vi "ImpedanceControl.vi"() -> ()   [LabVIEW 2018]
uses:
  <vilib>/Analysis/3filter.llb/Filter Passband Type.ctl
  <vilib>/DAQmx/write.llb/DAQmx Write (Analog DBL 1Chan 1Samp).vi
  <vilib>/DAQmx/read.llb/DAQmx Read (Analog 1D DBL NChan 1Samp).vi
  <vilib>/DAQmx/create/channels.llb/DAQmx Create Channel (AI-Voltage-Basic).vi
  <vilib>/DAQmx/create/channels.llb/DAQmx Create Channel (AO-Voltage-Basic).vi
  <vilib>/DAQmx/miscellaneous.llb/DAQmx Fill In Error Info.vi
  <vilib>/ptbypt/NI_PtbyPt.lvlib
  <vilib>/Analysis/NI_AALBase.lvlib
panel:
  out "Vel Measured":dbl(graph)
  out "Force Measurement":dbl(graph)
  in  "B":dbl min=0.0 step=0.01
  in  "K":dbl min=0.0 step=0.1
  in  "Wall Y/N":bool
  in  "Filter V y/n":bool
  in  "Filter P y/n":bool
  out "Output Voltage":dbl(graph)
  out "Position measurement":dbl(graph)
  in  "Gravity":bool
  in  "Friction":bool
  out "Measurements":dynamicdata(graph)
  in  "stop":bool
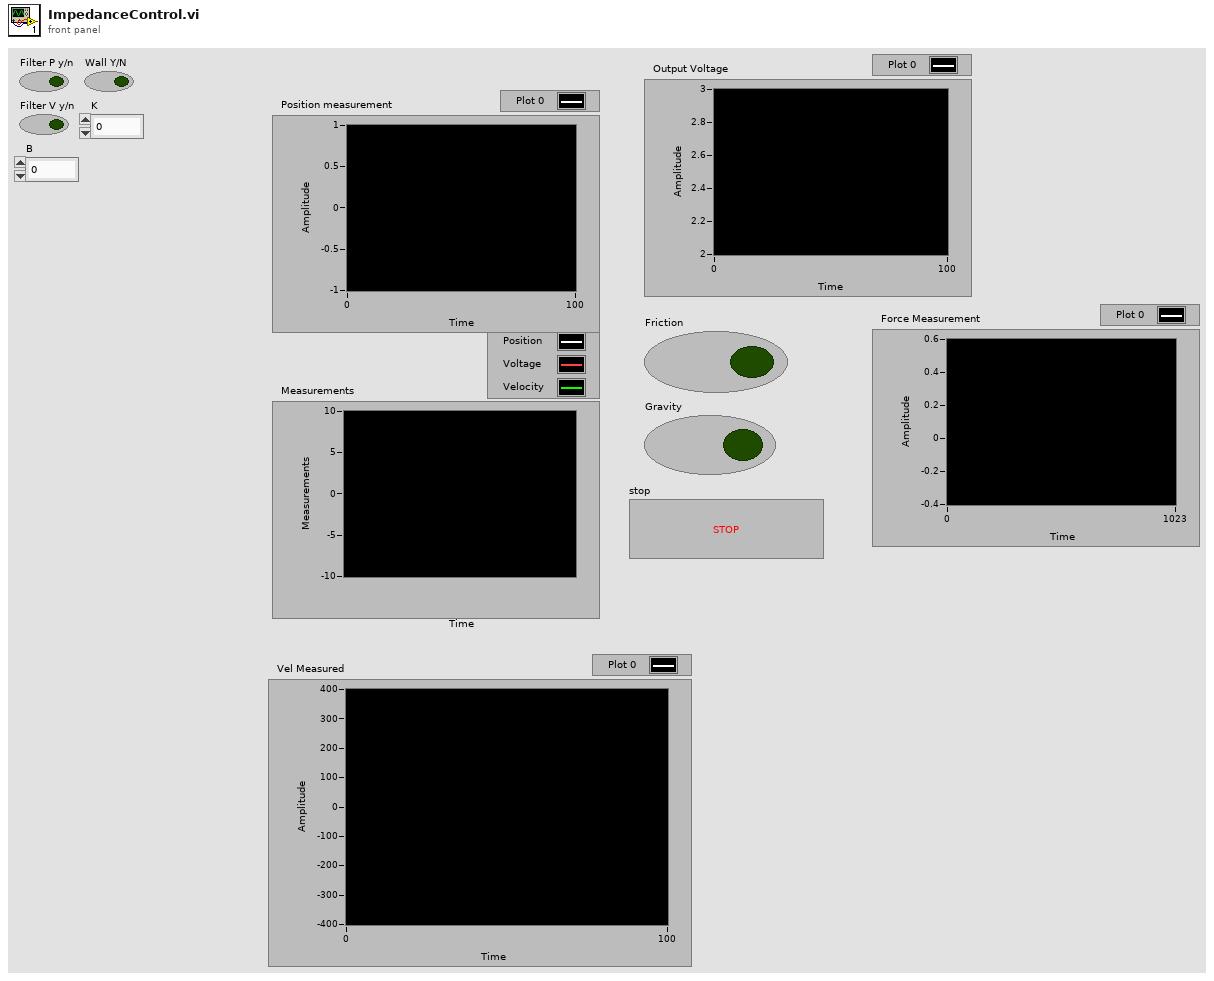
[diagram p1: front panel]
types:
  T1 = typedef "NI_AALBase.lvlib/Filter Passband Type.ctl" = enum32{"Lowpass", "Highpass", "Bandpass", "Bandstop"}
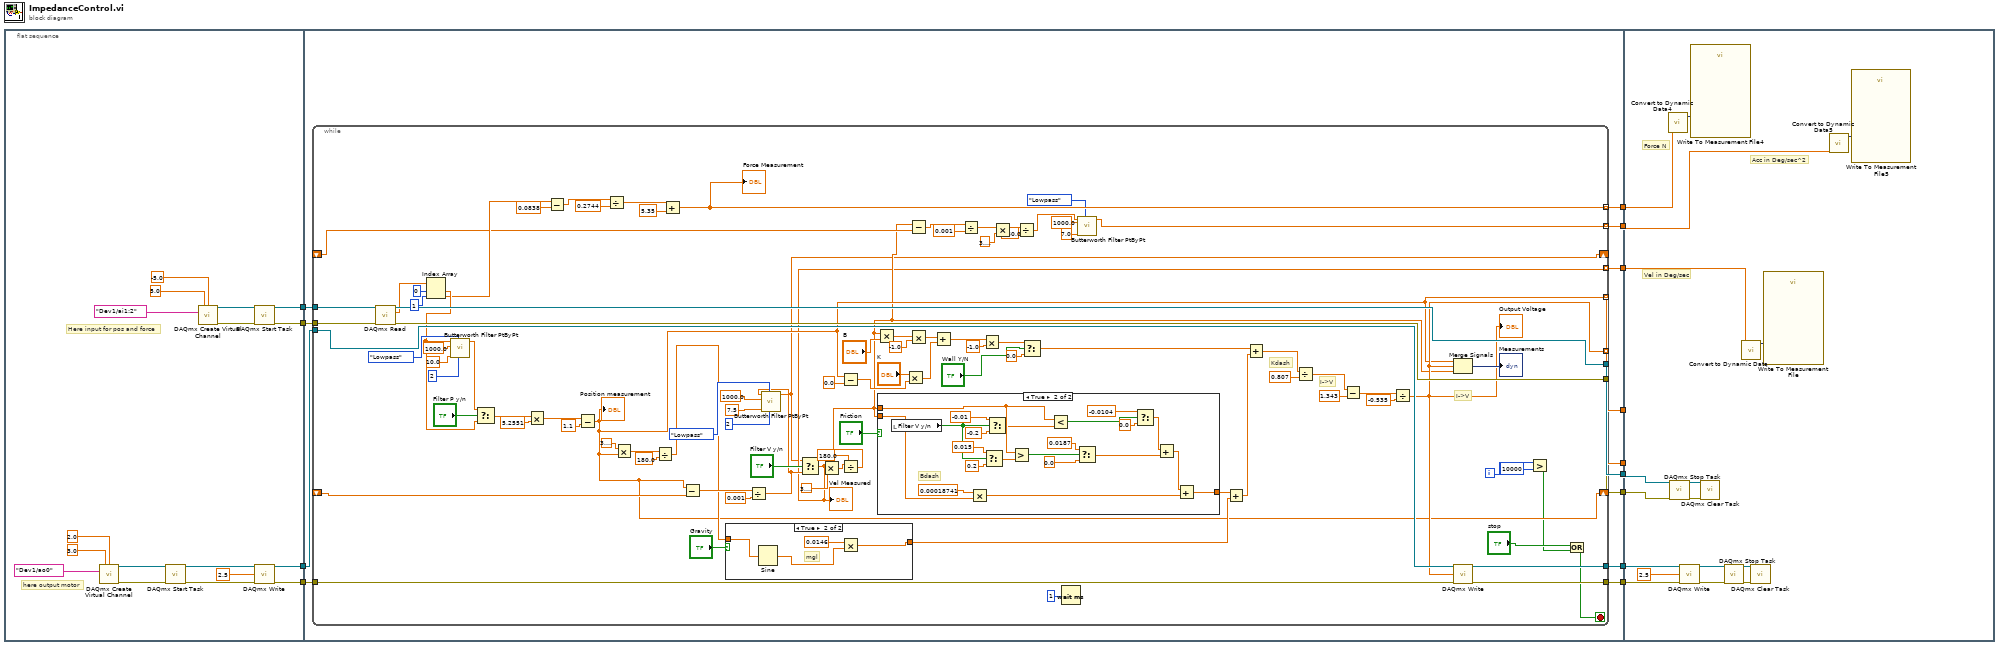
[diagram p0: block diagram]
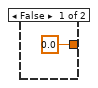
[diagram p2: hidden frame]
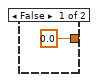
[diagram p3: hidden frame]
diagram:
  n1 = flat-sequence {
    tunnel: [w26] -> w12
    tunnel: [w25] -> w10
    tunnel: [w20] -> w9
    tunnel: [w18] -> w7
    tunnel: [w42] -> w13
    tunnel: w12 -> [w43]
    tunnel: [w40] -> w11
    tunnel: w10 -> [w41]
    tunnel: w9 -> [w39]
    tunnel: [w38] -> w8
    tunnel: w7 -> [w37]
    tunnel: [w36] -> w6
    tunnel: [w35] -> w5
    tunnel: [w34] -> w4
    tunnel: [w33] -> w3
    tunnel: [w32] -> w2
    tunnel: [w31] -> w1
    tunnel: w13 -> [w181]
    tunnel: w11 -> [w178]
    tunnel: w8 -> [w174]
    tunnel: w6 -> [w172]
    tunnel: w5 -> [_]
    tunnel: w4 -> [_]
    tunnel: w3 -> [w170]
    tunnel: w2 -> [w168]
    tunnel: w1 -> [w166]
    frame #0 {
      # "here output motor"
      # "Here input for pos and force"
      n2 = call-poly <vilib>:"DAQmx Create Virtual Channel.vi"("maximum value"=3.0, "minimum value"=2.0, "physical channels"=tag "Dev1/ao0") -> ("task out"=w30:refnum<k21>, "error out"=w29:errorcluster)  [unwired: 11 in]
      n3 = call <vilib>:"DAQmx Start Task.vi"("task/channels in"=w30, "error in"=w29) -> ("task out"=w28:refnum<k21>, "error out"=w27:errorcluster)  [unwired: 12 in]
      n4 = call-poly <vilib>:"DAQmx Create Virtual Channel.vi"("maximum value"=5.0, "minimum value"=-5.0, "physical channels"=tag "Dev1/ai1:2") -> ("task out"=w21:refnum<k21>, "error out"=w19:errorcluster)  [unwired: 11 in]
      n5 = call <vilib>:"DAQmx Start Task.vi"("task/channels in"=w21, "error in"=w19) -> ("task out"=w20:refnum<k21>, "error out"=w18:errorcluster)  [unwired: 12 in]
      n6 = call-poly <vilib>:"DAQmx Write.vi"("task/channels in"=w28, "data"=2.5, "error in"=w27) -> ("task out"=w26:refnum<k21>, "error out"=w25:errorcluster)  [unwired: 10 in, 1 out]
    }
    frame #1 {
      n7 = while {
        tunnel: w43 -> [w137]
        tunnel: [w136] -> w42
        tunnel: w41 -> [w135]
        tunnel: [w134] -> w40
        tunnel: w39 -> [w133]
        tunnel: [w132] -> w38
        tunnel: w37 -> [w131]
        tunnel: [w130] -> w36
        tunnel: [w65] -> w35 mode=indexing
        tunnel: [w101] -> w34 mode=indexing
        shift-right: [w65] -> _
        shift-left: _ -> [w122]
        tunnel: [w64] -> w33 mode=indexing
        shift-right: [w49] -> _
        shift-left: _ -> [w74]
        tunnel: [w53] -> w32 mode=indexing
        tunnel: [w59] -> w31 mode=indexing
        i -> [w57]
        stop <- w54 stop-if-true
        # "I->V"
        # "I->V"
        # "Kdash"
        n8 = call-poly <vilib>:"DAQmx Read.vi"("task/channels in"=w133, "error in"=w131) -> ("task out"=w132:refnum<k21>, "data"=w84:dbl[], "error out"=w130:errorcluster)  [unwired: 11 in]
        n9 = Index Array(array=w84, index #1=0 ("index"), index #2=1 ("index")) -> (element #1=w81:dbl, element #2=w80:dbl)
        n10 = call <vilib>:"Butterworth Filter PtByPt.vi"("order"=2, "filter type"=Filter_Passband_Type."Lowpass", "low cutoff freq: fl"=10.0, "sampling freq: fs"=1000.0, "x"=w81) -> ("Filtered x"=w99:dbl)  [unwired: 4 in, 1 out]
        n11 = Select(t=w99, s="Filter P y/n", f=w81) -> (s? t:f=w93:dbl)
        n12 = Multiply(x=w93, y=5.2551) -> (x*y=w123:dbl)
        n13 = Subtract(x=w80, y=0.0838) -> (x-y=w78:dbl)
        n14 = Subtract(x=w123, y=1.1) -> (x-y=w65:dbl)
        "Position measurement" <- w65
        n15 = Divide(x=w78, y=0.2744) -> (x/y=w76:dbl)
        n16 = Multiply(x=3.141592653589793, y=w65) -> (x*y=w105:dbl)
        n17 = Divide(x=w105, y=180.0) -> (x/y=w70:dbl)
        n18 = Add(x=w76, y=5.35) -> (x+y=w64:dbl)
        "Force Measurement" <- w64
        n19 = Subtract(x=w65, y=w122) -> (x-y=w116:dbl)
        n20 = case shown="True" "Gravity" {
          tunnel: [0.0 w164] -> w117
          tunnel: w70 -> [_ w161]
          frame False {
          }
          frame True {
            # "mgl"
            n21 = Sine(x=w161) -> (sin(x)=w163:dbl)
            n22 = Multiply(x=0.0146, y=w163) -> (x*y=w164:dbl)
          }
        }
        n23 = Divide(x=w116, y=0.001) -> (x/y=w85:dbl)
        n24 = call <vilib>:"Butterworth Filter PtByPt.vi"("order"=2, "filter type"=Filter_Passband_Type."Lowpass", "low cutoff freq: fl"=7.5, "sampling freq: fs"=1000.0, "x"=w85) -> ("Filtered x"=w49:dbl)  [unwired: 4 in, 1 out]
        n25 = Select(t=w49, s="Filter V y/n", f=w85) -> (s? t:f=w59:dbl)
        "Vel Measured" <- w59
        n26 = Multiply(x=w59, y=3.141592653589793) -> (x*y=w62:dbl)
        n27 = Subtract(x=w65, y=0.0) -> (x-y=w89:dbl)
        n28 = Divide(x=w62, y=180.0) -> (x/y=w60:dbl)
        n29 = Multiply(x=w60, y="B") -> (x*y=w68:dbl)
        n30 = case shown="True" "Friction" {
          tunnel: w60 -> [_ w159]
          tunnel: [0.0 w150] -> w118
          tunnel: w60 -> [_ w149]
          frame False {
          }
          frame True {
            # "Bdash"
            n31 = local read "Filter V y/n"() -> (w146:bool)
            n32 = Multiply(x=0.00018741, y=w159) -> (x*y=w151:dbl)
            n33 = Select(t=0.015, s=w146, f=0.2) -> (s? t:f=w155:dbl)
            n34 = Select(t=-0.01, s=w146, f=-0.2) -> (s? t:f=w145:dbl)
            n35 = Greater?(x=w149, y=w155) -> (0:w154:bool)
            n36 = Less?(x=w149, y=w145) -> (x < y?=w142:bool)
            n37 = Select(t=0.0187, s=w154, f=0.0) -> (s? t:f=w140:dbl)
            n38 = Select(t=-0.0104, s=w142, f=0.0) -> (s? t:f=w141:dbl)
            n39 = Add(x=w141, y=w140) -> (x+y=w139:dbl)
            n40 = Add(x=w139, y=w151) -> (x+y=w150:dbl)
          }
        }
        n41 = Multiply(x="K", y=w89) -> (x*y=w91:dbl)
        n42 = Subtract(x=w60, y=w74) -> (x-y=w73:dbl)
        n43 = Multiply(x=w68, y=-1.0) -> (x*y=w66:dbl)
        n44 = Add(x=w66, y=w91) -> (x+y=w88:dbl)
        n45 = Divide(x=w73, y=0.001) -> (x/y=w47:dbl)
        n46 = Multiply(x=w88, y=-1.0) -> (x*y=w86:dbl)
        n47 = Multiply(x=w47, y=3.141592653589793) -> (x*y=w48:dbl)
        n48 = Divide(x=w48, y=180.0) -> (x/y=w44:dbl)
        n49 = Select(t=w86, s="Wall Y/N", f=0.0) -> (s? t:f=w95:dbl)
        n50 = Wait (ms)(milliseconds to wait=u32 1) -> ()  [unwired: 1 out]
        n51 = call <vilib>:"Butterworth Filter PtByPt.vi"("filter type"=Filter_Passband_Type."Lowpass", "low cutoff freq: fl"=7.0, "sampling freq: fs"=1000.0, "x"=w44) -> ("Filtered x"=w53:dbl)  [unwired: 5 in, 1 out]
        n52 = Add(x=w118, y=w117) -> (x+y=w97:dbl)
        n53 = Add(x=w95, y=w97) -> (x+y=w96:dbl)
        n54 = Divide(x=w96, y=0.807) -> (x/y=w119:dbl)
        n55 = Subtract(x=w119, y=1.343) -> (x-y=w120:dbl)
        n56 = Divide(x=w120, y=-0.535) -> (x/y=w101:dbl)
        "Output Voltage" <- w101
        n57 = Merge Signals(w65, w101, w60) -> (→"Measurements":dynamicdata)
        n58 = call-poly <vilib>:"DAQmx Write.vi"("task/channels in"=w137, "data"=w101, "error in"=w135) -> ("task out"=w136:refnum<k21>, "error out"=w134:errorcluster)  [unwired: 10 in, 1 out]
        n59 = Greater?(x=w57, y=10000) -> (0:w55:bool)
        n60 = Or(x="stop", y=w55) -> (x .or. y?=w54:bool)
      }
    }
    frame #2 {
      # "Force N"
      # "Acc in Deg/sec^2"
      # "Vel in Deg/sec"
      n61 = call "Convert to Dynamic Data4"("Array"=w170) -> ("Dynamic Data Type"=w169:dynamicdata)  [unwired: 3 in]
      n62 = call <vilib>:"DAQmx Stop Task.vi"("task/channels in"=w174, "error in"=w172) -> ("task out"=w173:refnum<k21>, "error out"=w171:errorcluster)  [unwired: 12 in]
      n63 = call-poly <vilib>:"DAQmx Write.vi"("task/channels in"=w181, "data"=2.5, "error in"=w178) -> ("task out"=w180:refnum<k21>, "error out"=w177:errorcluster)  [unwired: 10 in, 1 out]
      n64 = call "Write To Measurement File4"("Signals"=w169) -> ()  [unwired: 16 in, 3 out]
      n65 = call <vilib>:"DAQmx Clear Task.vi"("task in"=w173, "error in"=w171) -> ()  [unwired: 13 in, 1 out]
      n66 = call <vilib>:"DAQmx Stop Task.vi"("task/channels in"=w180, "error in"=w177) -> ("task out"=w179:refnum<k21>, "error out"=w176:errorcluster)  [unwired: 12 in]
      n67 = call "Convert to Dynamic Data"("Array"=w166) -> ("Dynamic Data Type"=w165:dynamicdata)  [unwired: 3 in]
      n68 = call <vilib>:"DAQmx Clear Task.vi"("task in"=w179, "error in"=w176) -> ()  [unwired: 13 in, 1 out]
      n69 = call "Write To Measurement File"("Signals"=w165) -> ()  [unwired: 16 in, 3 out]
      n70 = call "Convert to Dynamic Data5"("Array"=w168) -> ("Dynamic Data Type"=w167:dynamicdata)  [unwired: 3 in]
      n71 = call "Write To Measurement File5"("Signals"=w167) -> ()  [unwired: 16 in, 3 out]
    }
  }
